vi "Delete empty element from array.vi"(0 "Array In":string[](array[string])) -> (20 "Array out":string[](array[string]))   [LabVIEW 2011]
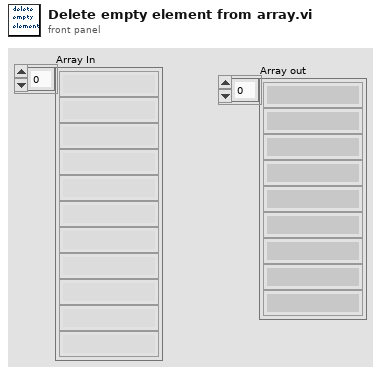
[diagram p1: front panel]
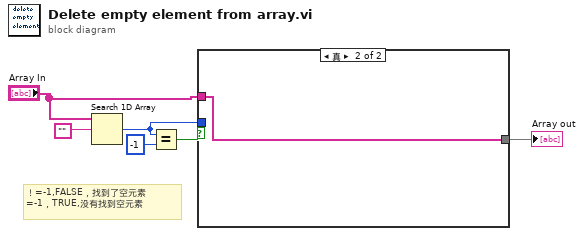
[diagram p0: block diagram]
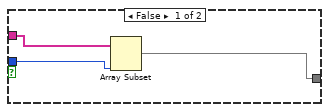
[diagram p2: hidden frame]
diagram:
  # "！=-1,FALSE，找到了空元素\n=-1，TRUE,没有找到空元素"
  n1 = Search 1D Array(1D array="Array In", element="") -> (index of element=w1:i32)  [unwired: 1 in]
  n2 = Equal?(x=w1, y=-1) -> (x = y?=w4:bool)
  n3 = case shown="真" w4 {
    tunnel: "Array In" -> [w9 w10]
    tunnel: [w7 w10] -> w2
    tunnel: w1 -> [w8 _]
    frame False {
      n4 = Array Subset(array=w9, length=w8) -> (w7:string[])  [unwired: 1 in]
    }
    frame True {
    }
  }
  "Array out" <- w2
